vi "! SI Image TCP-IP Client 4.vi"(0 "TCP/IP Address":string="Localhost") -> ()   [LabVIEW 2015]
doc: "This is a robust TCP/IP receiver (client) vi written to work with the transmitter (server) example. This routine is designed to work in the following way:\n\n1. Runs 24/7 and waits to the server to attach to the port and starts to receive data.\n2. Senses when there is not data - but the server is running - shows that server is attached, but is waiting for data.\n3. Senses when there is no server and polls the TCP/IP port for the server to attach. Attaches to the server and begins receipt of data when server begins sending.\n3. Will not stop, quit or error unless you press the STOP button.\n\nNotes: For sub-VI use you'll need to make 2 possbile changes:\nSince this runs all the time - this will halt execution when used as a sub-VI unless \n1. Add Global Vars inside this routine and run it in a seperate loop.\n2. Simply wire the STOP button down so it only runs once.\n\n\nWritten by: Jack Hamilton\nHamilton2@aol.com\nEngineering Consulting\nLab-Useful: LabVIEW tips, Tricks and downloads\nHttp://www.lanset.com/salient1\n714-839-6375 Office (Southern California)\n\nPermission by author for free distribution"
uses:
  Client Acquisition Mode Menu.ctl
  Frame Mode 1.ctl
  CCD Format.ctl
panel:
  in  "index 3":i32=2
  in  "index 2":i32=1
  in  "index 1":i32
  in  "Set CCD Format":bool
  in  "Readout Mode":u8(ring) items=["Mode 0", "Mode 1"]
  in  "CCD Format Parameters":T1={"Serial Origin"=50, "Serial Length"=512, "Serial Binning"=1, "Parallel Origin"=0, "Parallel Length"=1024, "Parallel Binning"=1} {"Parallel Binning" min=1 max=5000 step=1; "Parallel Length" min=0 max=65535 step=1; "Parallel Origin" min=0 max=9000 step=1; "Serial Binning" min=1 max=5000 step=1; "Serial Length" min=0 max=65535 step=1; "Serial Origin" min=0 max=9000 step=1}
  in  "Save":bool
  in  "Frames":i32=1 min=1 step=1
  in  "Frame Mode":T2 items=["Single Frame Buffer", "Multiple Frame Buffer"]
  in  "Acq Mode":T3 caption="Acquisition Mode"
  in  "# to Average":u32=2 caption="of"
  out "Acquiring":u32
  in  "Save As":u16(ring) items=["U16 FITS", "I16 FITS", "I32 FITS", "SGL FITS", "U16 TIFF", "I16 TIFF", "I32 TIFF", "SGL TIFF"]
  out "P Len":i32
  out "S Len":i32
  out "Vacuum Pressure":sgl format="%.3f"
  out "Backplate Temp.":sgl format="%.1f"
  out "CCD Temp.":sgl format="%.1f"
  out "Camera Status [ ]":sgl[](array[numeric])
  out "Image Header":string
  in  "Function":T4(ring)
  in  "Perform Function":bool
  out "Function #":u16
  out "Packet\nError code":i32
  out "Image":sgl[][](graph)
  in  "RO Done":bool
  out "% Complete":u16(slide) caption="% Readout" scale=0.0..100.0
  out "% Exposure":u16(slide) scale=0.0..100.0
  in  "File Name":string
  out "TCP/IP ID":refnum<k5>
  in  "TCP/IP Mode":u16(ring)=1 items=["Retrieve Image Buffer", "Acquire and transfer to client", "Acquire and hold in Server Image Buffer", "Acquire, transfer to client and save to Server's disk", "Acquire, save to Server's disk and hold in Server Image Buffer"]
  in  "Exposure Time":dbl=0.1 min=0.0 format="%.3t"
  in  "Acq 1 Type":u16(ring) items=["Light Exposure", "Dark Exposure", "Test Image", "Triggered Acq.", "TDI Internal Paced", "TDI External Paced"]
  in  "Acquire":bool
  in  "Display Style":i32(ring)=3 items=["Normal String", "\\ Codes", "Password", "Hexdump"]
  out "Read String":string
  in  "Stop":bool
  out "Connection Status":bool
  out "Error out":errorcluster
  in  "Port":u16=2055
  # "TCP/IP Settings"
  # "Connection Status"
  # "(Use 'Localhost' for same machine)"
  # "Parallel"
  # "Serial"
  # "Origin"
  # "Length"
  # "Binning"
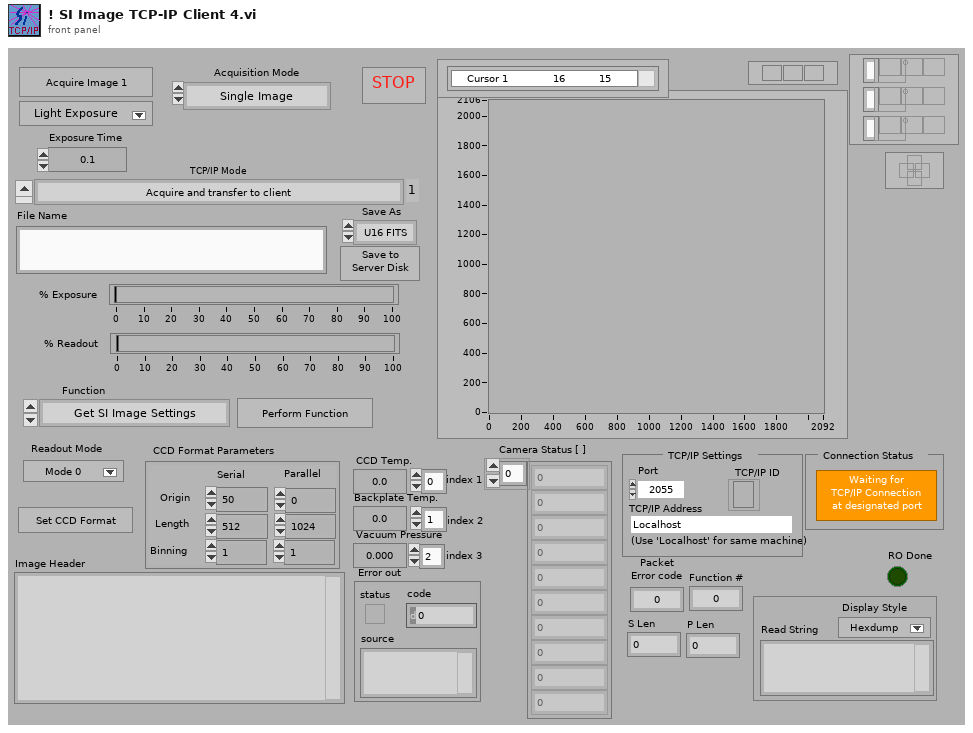
[diagram p1: front panel]
types:
  T1 = typedef "CCD Format.ctl" = cluster{"Serial Origin":i32, "Serial Length":i32, "Serial Binning":i32, "Parallel Origin":i32, "Parallel Length":i32, "Parallel Binning":i32}
  T2 = typedef "Frame Mode 1.ctl" = i32
  T3 = typedef "Client Acquisition Mode Menu.ctl" = enum16{"Single Image", "Average Images", "Multiple Frames"}
  T4 = enum16{"Get SI Image Settings", "Get Camera Status", "Get Image 1 Header", "Get Image 2 Header"}
  T5 = cluster{"% Exp.":u16, "%Readout":u16, "Relative Pos.":u32, "Acquiring":dbl}
  T6 = typedef "TCP-IP Image Packet.ctl" = cluster{"Image ID":u16, "Image Type":u16, "Serial Length":u16, "Parallel Length":u16, "# of Packets":u16, "Packet #":u16, "Offset":u32, "Image Bytes":u32, "Image Data $":string}
  T7 = typedef "SI Image Settings 1.ctl" = cluster{"Exp. Time":u32, "# of Modes":u8, "Mode #":u8, "Avg N Images":u32, "Frames":u32, "Acq. Mode":u16, "Acq. Type":u16, "Serial Origin":i32, "Serial Length":i32, "Serial Binning":i32, "Parallel Origin":i32, "Parallel Length":i32, "Parallel Binning":i32}
  T8 = cluster{"Serial Origin":i32, "Serial Length":i32, "Serial Binning":i32, "Parallel Origin":i32, "Parallel Length":i32, "Parallel Binning":i32}
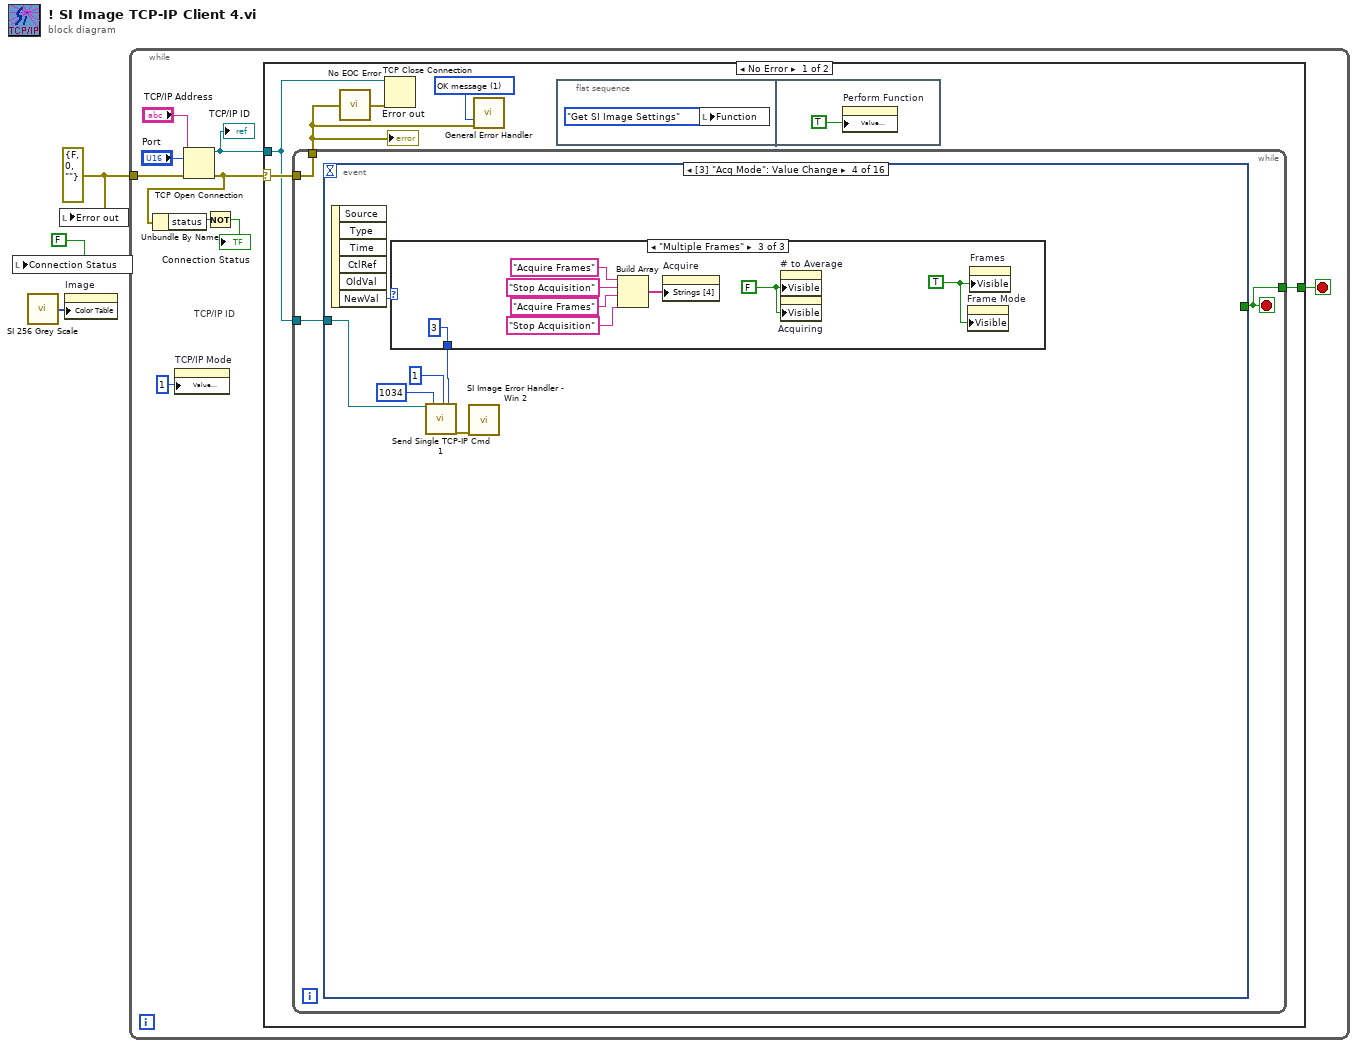
[diagram p0: block diagram]
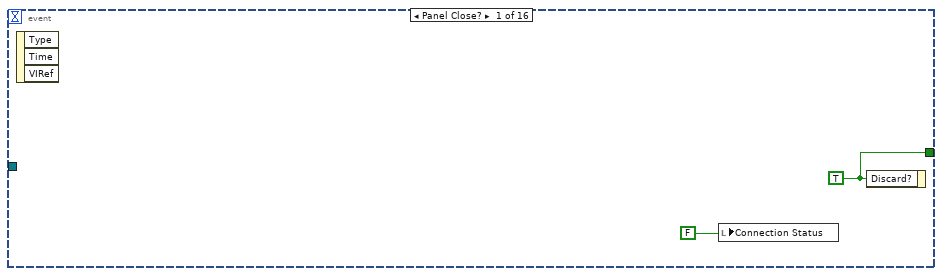
[diagram p2: hidden frame]
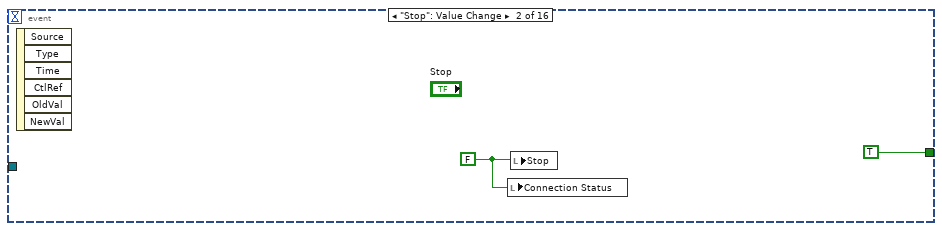
[diagram p3: hidden frame]
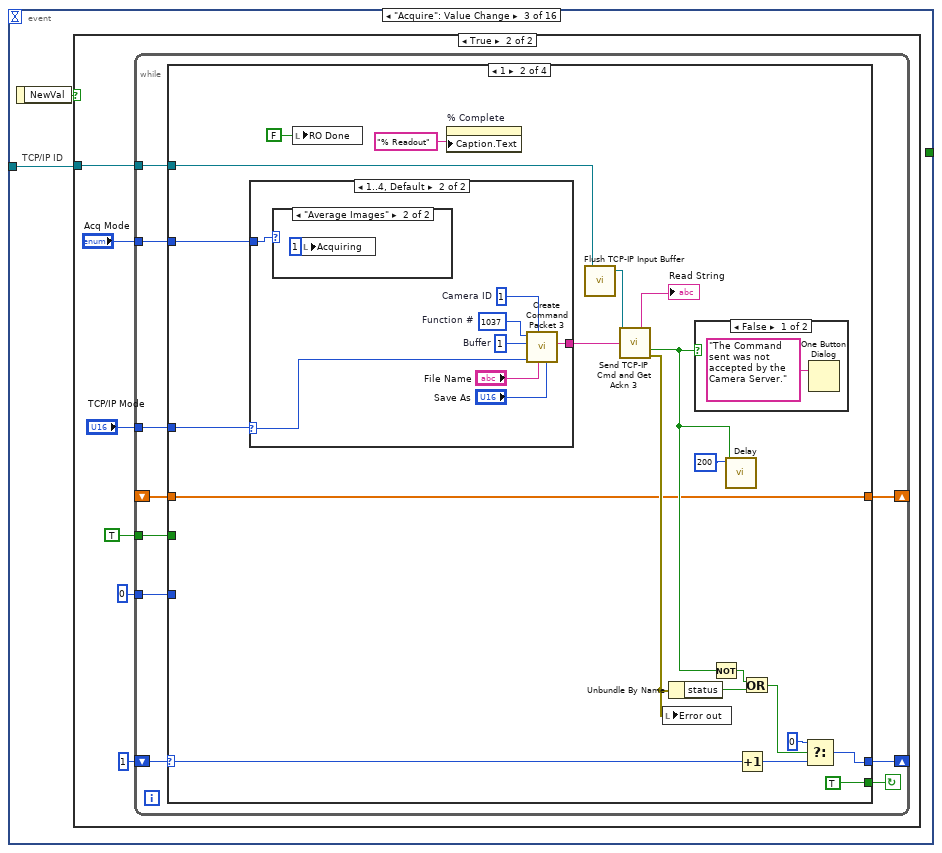
[diagram p4: hidden frame]
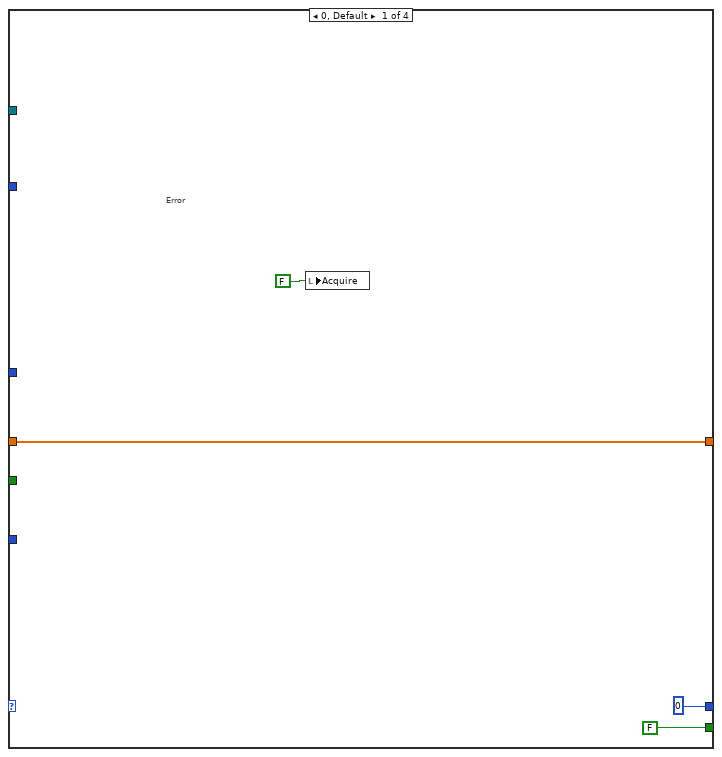
[diagram p6: hidden frame]
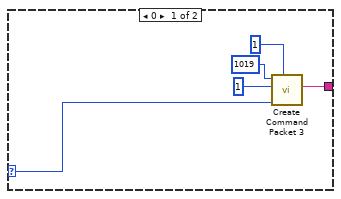
[diagram p7: hidden frame]
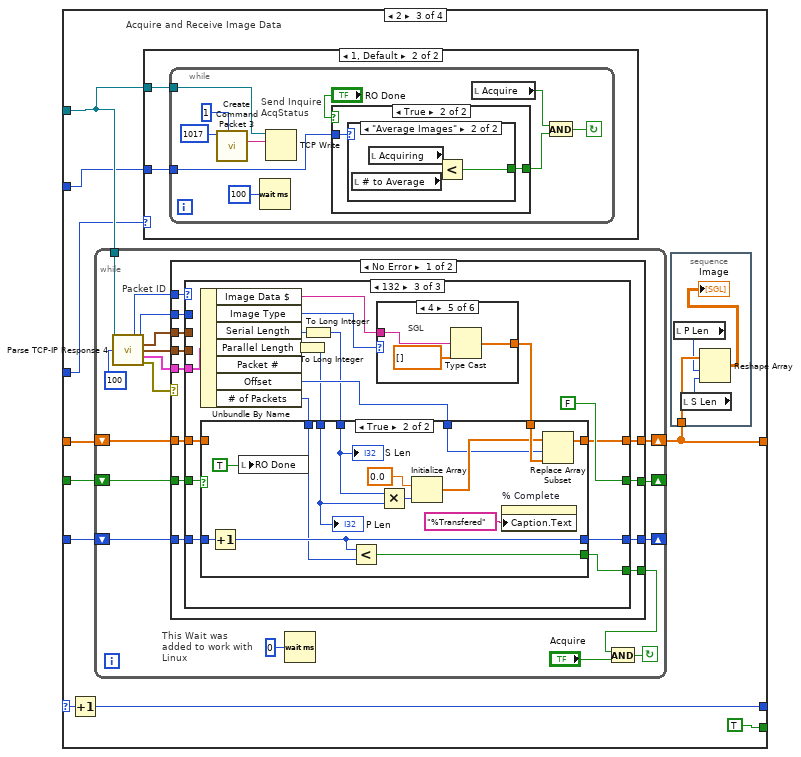
[diagram p10: hidden frame]
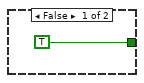
[diagram p12: hidden frame]
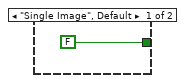
[diagram p13: hidden frame]
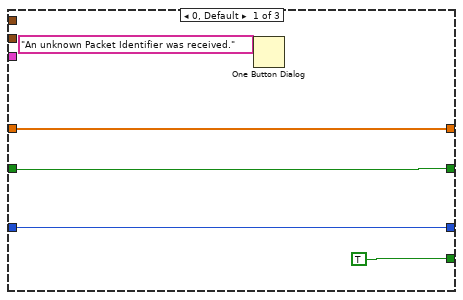
[diagram p14: hidden frame]
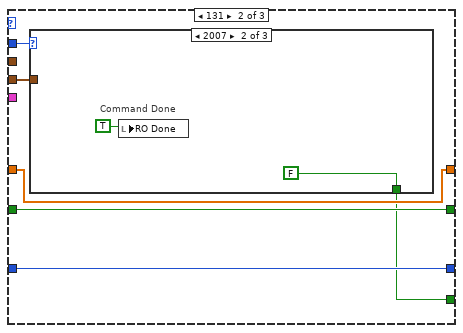
[diagram p15: hidden frame]
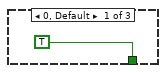
[diagram p16: hidden frame]
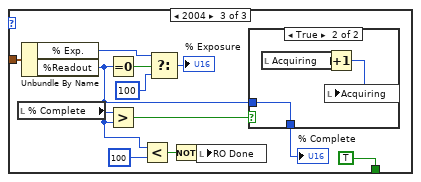
[diagram p17: hidden frame]
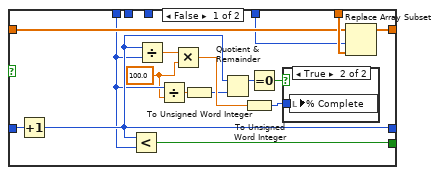
[diagram p19: hidden frame]
diagram:
  w3 = errorcluster {"status"=FALSE, "code"=0, "source"=""} ("error in (no error)")
  n1 = local write "Connection Status"(FALSE ("stop")) -> ()
  n2 = call "SI 256 Grey Scale.vi"() -> (w1:u32[])
  n3 = local write "Error out"(w3) -> ()
  n4 = property on="Image" class="IntGraph (strict)"("Color Table"=w1) -> ()  [unwired: 2 in, 2 out]
  n5 = while {
    tunnel: w3 -> [w7]
    stop <- w8 stop-if-true
    # "TCP/IP ID"
    n6 = property on="TCP/IP Mode" class="Ring (strict)"("Value (Signaling)"=u16 1) -> ()  [unwired: 2 in, 2 out]
    n7 = TCP Open Connection(address="TCP/IP Address", remote port or service name="Port", error in (no error)=w7) -> (connection ID=w12:refnum<k5>, error out=w9:errorcluster)  [unwired: 2 in]
    "TCP/IP ID" <- w12
    n8 = Unbundle By Name(w9) -> ("status"=w10:bool)
    n9 = Not(x=w10) -> (.not. x?=→"Connection Status":bool)
    n10 = case shown="No Error" w9 {
      selector: w9 -> [w17 _]
      tunnel: w12 -> [w14 _]
      tunnel: [w16 w540] -> w8
      frame No Error {
        w18 = u16 1 items=["no dialog", "OK message", "continue or stop message"] ("type of dialog (OK msg:1)")
        n11 = while {
          tunnel: [w22] -> w16
          tunnel: [w23] -> w13
          tunnel: w17 -> [w23]
          tunnel: w14 -> [w21]
          stop <- w22 stop-if-true
          n12 = event shown="[3] \"Acq Mode\": Value Change" {
            selector: _ -> [_ _ _ _ _ _ _ _ _ _ _ _ _ _ _ _]
            dyn-events: _ -> [_ _ _ _ _ _ _ _ _ _ _ _ _ _ _ _]
            timeout: _ -> [_ _ _ _ _ _ _ _ _ _ _ _ _ _ _ _]
            tunnel: [w25 TRUE _ _ _ _ _ _ _ _ _ _ _ _ _ _] -> w22
            tunnel: w21 -> [_ _ w28 w295 w330 w336 w344 w349 w354 w360 w366 w372 _ w415 _ _]
            event Panel Close? {
              w25 = TRUE ("Discard?")
              n13 = event-data() -> ()  [unwired: 1 in, 3 out]
              n14 = local write "Connection Status"(FALSE ("stop")) -> ()
              n15 = event-data("Discard?"=w25) -> ()  [unwired: 1 in, 1 out]
            }
            event "Stop": Value Change {
              w26 = FALSE ("Stop")
              n16 = event-data() -> ()  [unwired: 1 in, 6 out]
              n17 = local write "Connection Status"(w26) -> ()
              n18 = local write "Stop"(w26) -> ()
            }
            event "Acquire": Value Change {
              # "TCP/IP ID"
              n19 = event-data() -> ("NewVal"=w29:bool)  [unwired: 1 in]
              n20 = case shown="True" w29 {
                tunnel: w28 -> [_ w34]
                frame False {
                }
                frame True {
                  n21 = while {
                    tunnel: u16 0 -> [w37]
                    tunnel: TRUE -> [w38]
                    shift-left: _ -> [w40]
                    shift-right: [w39] -> _
                    tunnel: w34 -> [w41]
                    tunnel: "TCP/IP Mode" -> [w42]
                    shift-left: 1 -> [w45]
                    shift-right: [w44] -> _
                    tunnel: "Acq Mode" -> [w36]
                    stop <- w43 continue-if-true
                    n22 = case shown="1" w45 {
                      selector: w45 -> [_ w69 w93 w268]
                      tunnel: [0 w61 w94 w268] -> w44
                      tunnel: [FALSE TRUE TRUE w263] -> w43
                      tunnel: w42 -> [_ w55 w85 w266]
                      tunnel: w41 -> [_ w67 w91 w267]
                      tunnel: w40 -> [w46 w51 w90 w262]
                      tunnel: [w46 w51 w87 w262] -> w39
                      tunnel: w38 -> [_ _ w89 _]
                      tunnel: w37 -> [_ _ w88 _]
                      tunnel: w36 -> [_ w50 w86 w261]
                      frame 0, Default {
                        # "Error"
                        n23 = local write "Acquire"(FALSE) -> ()
                      }
                      frame 1 {
                        n24 = case shown="1..4, Default" w55 {
                          selector: w55 -> [w71 w78]
                          tunnel: [w72 w80] -> w65
                          tunnel: w50 -> [_ w75]
                          frame 0 {
                            n25 = call "Create Command Packet 3.vi"("Camera ID (1)"=u8 1 ("Camera ID"), "Mode"=w71, "Buffer/Avg #/Frames"=u16 1 ("Buffer #"), "Function #"=u16 1019) -> ("Cmd Packet"=w72:string)  [unwired: 7 in]
                          }
                          frame 1..4, Default {
                            w82 = u16 1037  # Function #
                            w79 = u32 1  # Buffer
                            w81 = u8 1  # Camera ID
                            n26 = case shown="\"Average Images\"" w75 {
                              frame "Single Image", Default {
                              }
                              frame "Average Images" {
                                n27 = local write "Acquiring"(u32 1 ("Acquiring")) -> ()
                              }
                            }
                            n28 = call "Create Command Packet 3.vi"("Save As"="Save As", "File Name"="File Name", "Camera ID (1)"=w81, "Mode"=w78, "Buffer/Avg #/Frames"=w79, "Function #"=w82) -> ("Cmd Packet"=w80:string)  [unwired: 5 in]
                          }
                        }
                        n29 = local write "RO Done"(FALSE ("RO Done")) -> ()
                        n30 = property on="% Complete" class="Slide (strict)"("Caption.Text"="% Readout") -> ()  [unwired: 2 in, 2 out]
                        n31 = call "Flush TCP-IP Input Buffer.vi"("TCP/IP ID"=w67) -> ("TCP/IP ID Out"=w66:refnum<k5>)  [unwired: 4 in]
                        n32 = call "Send TCP-IP Cmd and Get Ackn 3.vi"("TCP/IP ID In"=w66, "Cmd Packet"=w65) -> ("Read String"=→"Read String":string, "Accepted Flag"=w57:bool, "error out"=w52:errorcluster)  [unwired: 7 in, 4 out]
                        n33 = local write "Error out"(w52) -> ()
                        n34 = Unbundle By Name(w52) -> ("status"=w64:bool)
                        n35 = case shown="False" w57 {
                          frame False {
                            n36 = One Button Dialog(message="The Command sent was not accepted by the Camera Server.") -> ()  [unwired: 1 in, 1 out]
                          }
                          frame True {
                          }
                        }
                        n37 = Not(x=w57) -> (.not. x?=w59:bool)
                        n38 = call "Delay.vi"("Boolean In"=w57, "milliseconds to wait (10)"=u32 200) -> ()  [unwired: 8 in, 2 out]
                        n39 = Increment(x=w69) -> (x+1=w63:i32)
                        n40 = Or(x=w59, y=w64) -> (x .or. y?=w60:bool)
                        n41 = Select(t=0, s=w60, f=w63) -> (s? t:f=w61:i32)
                      }
                      frame 2 {
                        # "Acquire and Receive Image Data"
                        n42 = Increment(x=w93) -> (x+1=w94:i32)
                        n43 = while {
                          shift-left: w88 -> [w119]
                          shift-right: [w118] -> _
                          shift-left: w89 -> [w121]
                          shift-right: [w120] -> _
                          shift-left: w90 -> [w122]
                          shift-right: [w116] -> w87
                          tunnel: w91 -> [w131]
                          stop <- w127 continue-if-true
                          # "This Wait was added to work with Linux"
                          # "Packet ID"
                          n44 = call "Parse TCP-IP Response 4.vi"("TCP/IP ID"=w131, "timeout ms (5000)"=100) -> ("Packet ID"=w130:u8, "Data Type"=w124:u16, "Command Done"=w129:cluster{"Function #":u16}, "Acq. Status"=w128:T5, "Image Packet"=w123:T6, "error out"=w125:errorcluster)  [unwired: 3 in, 5 out]
                          n45 = case shown="No Error" w125 {
                            selector: w125 -> [_ w246]
                            tunnel: w130 -> [w143 _]
                            tunnel: w129 -> [w142 _]
                            tunnel: w128 -> [w141 _]
                            tunnel: [w140 w247] -> w126
                            tunnel: w124 -> [w139 _]
                            tunnel: w123 -> [w138 _]
                            tunnel: w122 -> [w137 w250]
                            tunnel: [w136 w250] -> w116
                            tunnel: w121 -> [w135 w251]
                            tunnel: [w134 w251] -> w120
                            tunnel: w119 -> [w133 w249]
                            tunnel: [w132 w249] -> w118
                            frame No Error {
                              n46 = case shown="132" w143 {
                                tunnel: w142 -> [_ _ _]
                                tunnel: w141 -> [_ w154 _]
                                tunnel: [TRUE w149 w179] -> w140
                                tunnel: w139 -> [_ w151 _]
                                tunnel: w138 -> [_ _ w187]
                                tunnel: w137 -> [w144 w150 w178]
                                tunnel: [w144 w150 w182] -> w136
                                tunnel: w135 -> [w147 w153 w177]
                                tunnel: [w147 w153 FALSE] -> w134
                                tunnel: w133 -> [w146 w152 w181]
                                tunnel: [w146 w152 w180] -> w132
                                frame 0, Default {
                                n47 = One Button Dialog(message="An unknown Packet Identifier was received.") -> ()  [unwired: 1 in, 1 out]
                                }
                                frame 131 {
                                n48 = case shown="2007" w151 {
                                tunnel: w154 -> [_ _ w170]
                                tunnel: [TRUE FALSE TRUE] -> w149
                                frame 0, Default {
                                }
                                frame 2007 {
                                # "Command Done"
                                n49 = local write "RO Done"(TRUE) -> ()
                                }
                                frame 2004 {
                                n50 = local read "% Complete"() -> (w164:u16)
                                n51 = Unbundle By Name(w170) -> ("% Exp."=w159:u16, "%Readout"=w162:u16)
                                n52 = Equal To 0?(x=w162) -> (x = 0?=w161:bool)
                                n53 = Greater?(x=w164, y=w162) -> (0:w163:bool)
                                n54 = Less?(x=w162, y=u16 100) -> (x < y?=w168:bool)
                                n55 = Select(t=w159, s=w161, f=u16 100) -> (s? t:f=→"% Exposure":u16)
                                n56 = Not(x=w168) -> (.not. x?=w167:bool)
                                n57 = local write "RO Done"(w167) -> ()
                                n58 = case shown="True" w163 {
                                tunnel: [w171 w172] -> w165
                                tunnel: w162 -> [w171 w172]
                                frame False {
                                }
                                frame True {
                                n59 = local read "Acquiring"() -> (w173:u32)
                                n60 = Increment(x=w173) -> (x+1=w174:u32)
                                n61 = local write "Acquiring"(w174) -> ()
                                }
                                }
                                "% Complete" <- w165
                                }
                                }
                                }
                                frame 132 {
                                n62 = Unbundle By Name(w187) -> ("Image Data $"=w190:string, "Image Type"=w189:u16, "Serial Length"=w186:u16, "Parallel Length"=w185:u16, "Offset"=w184:u32, "# of Packets"=w188:u16)  [unwired: 1 out]
                                n63 = To Long Integer(number=w185) -> (32bit integer=w175:i32)
                                n64 = To Long Integer(number=w186) -> (32bit integer=w176:i32)
                                n65 = case shown="4" w189 {
                                tunnel: [w225 w228 w233 w236 w240 w243] -> w183
                                tunnel: w190 -> [w223 w227 w231 w235 w239 w242]
                                frame 0, Default {
                                # "U16"
                                n66 = Type Cast(type=u16[] [] ("Array Constant"), x=w223) -> (*(type *) &x=w226:u16[])
                                n67 = To Single Precision Float(number=w226) -> (single precision float=w225:sgl[])
                                }
                                frame 1 {
                                # "I16"
                                n68 = Type Cast(type=i16[] [] ("Array Constant"), x=w227) -> (*(type *) &x=w230:i16[])
                                n69 = To Single Precision Float(number=w230) -> (single precision float=w228:sgl[])
                                }
                                frame 2 {
                                # "U32"
                                n70 = Type Cast(type=u32[] [] ("Array Constant"), x=w231) -> (*(type *) &x=w234:u32[])
                                n71 = To Single Precision Float(number=w234) -> (single precision float=w233:sgl[])
                                }
                                frame 3 {
                                # "I32"
                                n72 = Type Cast(type=i32[] [] ("Array Constant"), x=w235) -> (*(type *) &x=w238:i32[])
                                n73 = To Single Precision Float(number=w238) -> (single precision float=w236:sgl[])
                                }
                                frame 4 {
                                # "SGL"
                                n74 = Type Cast(type=sgl[] [] ("Array Constant"), x=w239) -> (*(type *) &x=w240:sgl[])
                                }
                                frame 5 {
                                # "DBL"
                                n75 = Type Cast(type=dbl[] [] ("Array Constant"), x=w242) -> (*(type *) &x=w245:dbl[])
                                n76 = To Single Precision Float(number=w245) -> (single precision float=w243:sgl[])
                                }
                                }
                                n77 = case shown="True" w177 {
                                tunnel: w178 -> [w198 _]
                                tunnel: w176 -> [_ w210]
                                tunnel: w175 -> [_ w209]
                                tunnel: [w199 w221] -> w182
                                tunnel: w183 -> [w207 w220]
                                tunnel: w181 -> [w206 w218]
                                tunnel: [w196 w217] -> w180
                                tunnel: [w205 w216] -> w179
                                tunnel: w184 -> [w197 w213]
                                tunnel: w188 -> [w194 w212]
                                frame False {
                                w193 = 100.0 ("y")
                                n78 = Increment(x=w206) -> (x+1=w196:u16)
                                n79 = Less?(x=w196, y=w194) -> (x < y?=w205:bool)
                                n80 = Divide(x=w196, y=w194) -> (x/y=w201:dbl)
                                n81 = Divide(x=w194, y=w193) -> (x/y=w195:dbl)
                                n82 = Multiply(x=w201, y=w193) -> (x*y=w200:dbl)
                                n83 = To Unsigned Word Integer(number=w195) -> (unsigned 16bit integer=w192:u16)
                                n84 = Quotient & Remainder(x=w196, y=w192) -> (x-y*floor(x/y)=w204:u16)  [unwired: 1 out]
                                n85 = To Unsigned Word Integer(number=w200) -> (unsigned 16bit integer=w202:u16)
                                n86 = Equal To 0?(x=w204) -> (x = 0?=w203:bool)
                                n87 = case shown="True" w203 {
                                tunnel: w202 -> [_ w208]
                                frame False {
                                }
                                frame True {
                                n88 = local write "% Complete"(w208) -> ()
                                }
                                }
                                n89 = Replace Array Subset(array=w198, new element=w207, index=w197) -> (w199:sgl[])
                                }
                                frame True {
                                n90 = Increment(x=w218) -> (x+1=w217:u16)
                                n91 = local write "RO Done"(TRUE) -> ()
                                n92 = Less?(x=w217, y=w212) -> (x < y?=w216:bool)
                                n93 = Multiply(x=w210, y=w209) -> (x*y=w214:i32)
                                n94 = Initialize Array(sgl 0.0 ("Element Data"), w214) -> (w219:sgl[])
                                n95 = property on="% Complete" class="Slide (strict)"("Caption.Text"="%Transfered") -> ()  [unwired: 2 in, 2 out]
                                n96 = Replace Array Subset(array=w219, new element=w220, index=w213) -> (w221:sgl[])
                                "S Len" <- w210
                                "P Len" <- w209
                                }
                                }
                                }
                              }
                            }
                            frame Error {
                              n97 = Unbundle By Name(w246) -> ("code"=w248:i32)
                              n98 = case shown="0, Default" w248 {
                                tunnel: w246 -> [w255 _]
                                tunnel: [w253 TRUE] -> w247
                                frame 0, Default {
                                w253 = FALSE
                                n99 = call <vilib>:"Simple Error Handler.vi"("error source (\" \")"="There was an error in a TCP/IP read during an Image Acquisition.", "error in (no error)"=w255) -> ("error out"=w252:errorcluster)  [unwired: 3 in, 4 out]
                                n100 = local write "Error out"(w252) -> ()
                                n101 = local write "Acquire"(w253) -> ()
                                }
                                frame 56 {
                                # "Timeout -  Keep going"
                                }
                              }
                            }
                          }
                          n102 = Wait (ms)(milliseconds to wait=u32 0) -> ()  [unwired: 1 out]
                          n103 = And(x=w126, y="Acquire") -> (x .and. y?=w127:bool)
                        }
                        n104 = case shown="1, Default" w85 {
                          tunnel: w91 -> [_ w96]
                          tunnel: w86 -> [_ w95]
                          frame 0 {
                          }
                          frame 1, Default {
                            n105 = while {
                              tunnel: w96 -> [w103]
                              tunnel: w95 -> [w97]
                              stop <- w101 continue-if-true
                              # "Send Inquire\nAcqStatus"
                              n106 = call "Create Command Packet 3.vi"("Camera ID (1)"=u8 1 ("Camera ID"), "Function #"=u16 1017) -> ("Cmd Packet"=w104:string)  [unwired: 9 in]
                              n107 = Wait (ms)(milliseconds to wait=u32 100) -> ()  [unwired: 1 out]
                              n108 = TCP Write(connection ID=w103, data in=w104) -> ()  [unwired: 2 in, 3 out]
                              n109 = case shown="True" "RO Done" {
                                tunnel: [TRUE w109] -> w100
                                tunnel: w97 -> [_ w108]
                                frame False {
                                }
                                frame True {
                                n110 = case shown="\"Average Images\"" w108 {
                                tunnel: [FALSE w111] -> w109
                                frame "Single Image", Default {
                                }
                                frame "Average Images" {
                                n111 = local read "# to Average"() -> (w112:u32)
                                n112 = local read "Acquiring"() -> (w113:u32)
                                n113 = Less?(x=w113, y=w112) -> (x < y?=w111:bool)
                                }
                                }
                                }
                              }
                              n114 = local read "Acquire"() -> (w98:bool)
                              n115 = And(x=w98, y=w100) -> (x .and. y?=w101:bool)
                            }
                          }
                        }
                        n116 = stacked-sequence {
                          tunnel: w87 -> [w260]
                          frame #0 {
                            n117 = local read "P Len"() -> (w259:i32)
                            n118 = local read "S Len"() -> (w258:i32)
                            n119 = Reshape Array(w260, w259, w258) -> (→"Image":sgl[][])
                          }
                        }
                      }
                      frame 3 {
                        w263 = FALSE
                        n120 = case shown="1, Default" w266 {
                          selector: w266 -> [w270 w279 w293]
                          tunnel: w267 -> [_ w280 _]
                          tunnel: [w270 w279 w293] -> w264
                          tunnel: w261 -> [_ w273 _]
                          frame 0 {
                          }
                          frame 1, Default {
                            # "If Exposure was not 100%, acquisition was terminated so send TerminateAcquisition command."
                            n121 = Equal?(x=w273, y=Client_Acquisition_Mode_Menu."Average Images") -> (x = y?=w271:bool)
                            n122 = local read "# to Average"() -> (w277:u32)
                            n123 = local read "% Exposure"() -> (w282:u16)
                            n124 = local read "Acquiring"() -> (w278:u32)
                            n125 = Less?(x=w278, y=w277) -> (x < y?=w276:bool)
                            n126 = Less?(x=w282, y=u16 100) -> (x < y?=w275:bool)
                            n127 = Select(t=w276, s=w271, f=w275) -> (s? t:f=w274:bool)
                            n128 = case shown="True" w274 {
                              tunnel: w280 -> [_ w291]
                              frame False {
                              }
                              frame True {
                                n129 = call "Create Command Packet 3.vi"("Camera ID (1)"=u8 1 ("Camera ID"), "Function #"=u16 1018) -> ("Cmd Packet"=w289:string)  [unwired: 9 in]
                                n130 = call "Flush TCP-IP Input Buffer.vi"("TCP/IP ID"=w291) -> ("TCP/IP ID Out"=w285:refnum<k5>)  [unwired: 4 in]
                                n131 = TCP Write(connection ID=w285, data in=w289) -> (error out=w288:errorcluster)  [unwired: 2 in, 2 out]
                                n132 = call "Parse TCP-IP Response 4.vi"("TCP/IP ID"=w285, "error in (no error)"=w288) -> ("Packet Error Code"=→"Packet\nError code":i32, "Command Done"=w287:cluster{"Function #":u16}, "error out"=w283:errorcluster)  [unwired: 3 in, 8 out]
                                n133 = Unbundle By Name(w287) -> ("Function #"=→"Function #":u16)
                                n134 = local write "Error out"(w283) -> ()
                              }
                            }
                          }
                          frame 5 {
                          }
                        }
                        n135 = stacked-sequence {
                          tunnel: w264 -> [_]
                          frame #0 {
                            w269 = u16 0 ("% Exposure")
                            n136 = local write "% Exposure"(w269) -> ()
                            n137 = local write "% Complete"(w269) -> ()
                            "Acquiring" <- w269
                          }
                        }
                        n138 = property on="% Complete" class="Slide (strict)"("Caption.Text"="% Readout") -> ()  [unwired: 2 in, 2 out]
                        n139 = local write "Acquire"(w263) -> ()
                      }
                    }
                  }
                }
              }
            }
            event Value Change {
              n140 = event-data() -> ("NewVal"=w299:T3)  [unwired: 1 in, 5 out]
              n141 = case shown="\"Multiple Frames\"" w299 {
                selector: w299 -> [w301 w310 _]
                tunnel: [w300 w309 u8 3 ("Acq. Mode/Type/Buffer")] -> w294
                frame "Single Image", Default {
                  w302 = FALSE ("Visible")
                  w303 = FALSE ("Visible")
                  n142 = To Unsigned Byte Integer(number=w301) -> (unsigned 8bit integer=w300:u8)
                  n143 = Build Array("Acquire Image 1", "Stop Acquisition", "Acquire Image 1", "Stop Acquisition") -> (w304:string[])
                  n144 = property on="Acquire" class="Bool (strict)"("Strings [4]"=w304) -> ()  [unwired: 2 in, 2 out]
                  n145 = property on="# to Average" class="DigNum (strict)"("Visible"=w302) -> ()  [unwired: 2 in, 2 out]
                  n146 = property on="Acquiring" class="DigNum (strict)"("Visible"=w302) -> ()  [unwired: 2 in, 2 out]
                  n147 = property on="Frames" class="DigNum (strict)"("Visible"=w303) -> ()  [unwired: 2 in, 2 out]
                  n148 = property on="Frame Mode" class="Ring (strict)"("Visible"=w303) -> ()  [unwired: 2 in, 2 out]
                }
                frame "Average Images" {
                  w311 = TRUE ("Visible")
                  w312 = FALSE ("Visible")
                  n149 = To Unsigned Byte Integer(number=w310) -> (unsigned 8bit integer=w309:u8)
                  n150 = Build Array("Acquire Average", "Stop Acquisition", "Acquire Average", "Stop Acquisition") -> (w313:string[])
                  n151 = property on="Acquire" class="Bool (strict)"("Strings [4]"=w313) -> ()  [unwired: 2 in, 2 out]
                  n152 = property on="# to Average" class="DigNum (strict)"("Visible"=w311) -> ()  [unwired: 2 in, 2 out]
                  n153 = property on="Acquiring" class="DigNum (strict)"("Visible"=w311) -> ()  [unwired: 2 in, 2 out]
                  n154 = property on="Frame Mode" class="Ring (strict)"("Visible"=w312) -> ()  [unwired: 2 in, 2 out]
                  n155 = property on="Frames" class="DigNum (strict)"("Visible"=w312) -> ()  [unwired: 2 in, 2 out]
                }
                frame "Multiple Frames" {
                  w319 = FALSE ("Visible")
                  w320 = TRUE ("Visible")
                  n156 = Build Array("Acquire Frames", "Stop Acquisition", "Acquire Frames", "Stop Acquisition") -> (w321:string[])
                  n157 = property on="Acquire" class="Bool (strict)"("Strings [4]"=w321) -> ()  [unwired: 2 in, 2 out]
                  n158 = property on="# to Average" class="DigNum (strict)"("Visible"=w319) -> ()  [unwired: 2 in, 2 out]
                  n159 = property on="Acquiring" class="DigNum (strict)"("Visible"=w319) -> ()  [unwired: 2 in, 2 out]
                  n160 = property on="Frame Mode" class="Ring (strict)"("Visible"=w320) -> ()  [unwired: 2 in, 2 out]
                  n161 = property on="Frames" class="DigNum (strict)"("Visible"=w320) -> ()  [unwired: 2 in, 2 out]
                }
              }
              n162 = call "Send Single TCP-IP Cmd 1.vi"("TCP/IP ID"=w295, "Function #"=u16 1034, "Camera ID"=u8 1, "Acq. Mode/Type/Frame Mode/RO Mode #"=w294) -> ("Error Out"=w296:errorcluster)  [unwired: 12 in, 3 out]
              n163 = call "SI Image Error Handler - Win 2.vi"("error in (no error)"=w296) -> ()  [unwired: 4 in, 1 out]
            }
            event "Exposure Time": Value Change {
              # "ET in ms"
              n164 = event-data() -> ("NewVal"=w327:dbl)  [unwired: 1 in, 5 out]
              n165 = Multiply(x=w327, y=1000.0) -> (x*y=w328:dbl)
              n166 = To Unsigned Long Integer(number=w328) -> (unsigned 32bit integer=w326:u32)
              n167 = call "Send Single TCP-IP Cmd 1.vi"("TCP/IP ID"=w330, "Exposure Time (ms)"=w326, "Function #"=u16 1035, "Camera ID"=u8 1) -> ("Error Out"=w331:errorcluster)  [unwired: 12 in, 3 out]
              n168 = call "SI Image Error Handler - Win 2.vi"("error in (no error)"=w331) -> ()  [unwired: 4 in, 1 out]
            }
            event "Readout Mode": Value Change {
              n169 = event-data() -> ("NewVal"=w335:u8)  [unwired: 1 in, 3 out]
              n170 = call "Send Single TCP-IP Cmd 1.vi"("TCP/IP ID"=w336, "Function #"=u16 1042, "Camera ID"=u8 1, "Acq. Mode/Type/Frame Mode/RO Mode #"=w335) -> ("Error Out"=w337:errorcluster)  [unwired: 12 in, 3 out]
              n171 = call "SI Image Error Handler - Win 2.vi"("error in (no error)"=w337) -> ("error out"=w334:errorcluster)  [unwired: 4 in]
              n172 = flat-sequence {
                tunnel: w334 -> [_]
                frame #0 {
                  n173 = local write "Function"(T4."Get SI Image Settings" ("Function")) -> ()
                }
                frame #1 {
                  n174 = property on="Perform Function" class="Bool (strict)"("Value (Signaling)"=TRUE) -> ()  [unwired: 2 in, 2 out]
                }
              }
            }
            event "Acq 1 Type": Value Change {
              n175 = event-data() -> ("NewVal"=w343:u16)  [unwired: 1 in, 5 out]
              n176 = call "Send Single TCP-IP Cmd 1.vi"("TCP/IP ID"=w344, "Buffer/Avg #/Frames"=u16 1, "Function #"=u16 1036, "Camera ID"=u8 1, "Acq. Mode/Type/Frame Mode/RO Mode #"=w343) -> ("Error Out"=w345:errorcluster)  [unwired: 11 in, 3 out]
              n177 = call "SI Image Error Handler - Win 2.vi"("error in (no error)"=w345) -> ()  [unwired: 4 in, 1 out]
            }
            event Value Change {
              n178 = event-data() -> ("NewVal"=w348:T2)  [unwired: 1 in, 5 out]
              n179 = call "Send Single TCP-IP Cmd 1.vi"("TCP/IP ID"=w349, "Function #"=u16 1040, "Camera ID"=u8 1, "Acq. Mode/Type/Frame Mode/RO Mode #"=w348) -> ("Error Out"=w350:errorcluster)  [unwired: 12 in, 3 out]
              n180 = call "SI Image Error Handler - Win 2.vi"("error in (no error)"=w350) -> ()  [unwired: 4 in, 1 out]
            }
            event "Frames": Value Change {
              n181 = event-data() -> ("NewVal"=w353:i32)  [unwired: 1 in, 5 out]
              n182 = call "Send Single TCP-IP Cmd 1.vi"("TCP/IP ID"=w354, "Buffer/Avg #/Frames"=w353, "Function #"=u16 1039, "Camera ID"=u8 1) -> ("Error Out"=w355:errorcluster)  [unwired: 12 in, 3 out]
              n183 = call "SI Image Error Handler - Win 2.vi"("error in (no error)"=w355) -> ()  [unwired: 4 in, 1 out]
            }
            event "Set CCD Format": Value Change {
              n184 = event-data() -> ()  [unwired: 1 in, 6 out]
              n185 = call "Send Single TCP-IP Cmd 1.vi"("TCP/IP ID"=w360, "Function #"=u16 1043, "Camera ID"=u8 1, "CCD Format Parameters"="CCD Format Parameters") -> ("Error Out"=w361:errorcluster)  [unwired: 12 in, 3 out]
              n186 = call "SI Image Error Handler - Win 2.vi"("error in (no error)"=w361) -> ("error out"=w358:errorcluster)  [unwired: 4 in]
              n187 = stacked-sequence {
                tunnel: w358 -> [_]
                frame #0 {
                  n188 = local write "Set CCD Format"(FALSE ("Set CCD Format")) -> ()
                }
              }
            }
            event "# to Average": Value Change {
              n189 = event-data() -> ("NewVal"=w365:u32)  [unwired: 1 in, 5 out]
              n190 = call "Send Single TCP-IP Cmd 1.vi"("TCP/IP ID"=w366, "Buffer/Avg #/Frames"=w365, "Function #"=u16 1038, "Camera ID"=u8 1) -> ("Error Out"=w367:errorcluster)  [unwired: 12 in, 3 out]
              n191 = call "SI Image Error Handler - Win 2.vi"("error in (no error)"=w367) -> ()  [unwired: 4 in, 1 out]
            }
            event "Save": Value Change {
              n192 = event-data() -> ("NewVal"=w371:bool)  [unwired: 1 in, 5 out]
              n193 = case shown="True" w371 {
                tunnel: w372 -> [_ w378]
                tunnel: [_ w374] -> w370
                frame False {
                }
                frame True {
                  n194 = local read "File Name"() -> (w376:string)
                  n195 = local read "Save As"() -> (w375:u16)
                  n196 = call "Send Single TCP-IP Cmd 1.vi"("TCP/IP ID"=w378, "Buffer/Avg #/Frames"=u16 1, "Function #"=u16 1031, "File Name"=w376, "Camera ID"=u8 1, "Save As"=w375) -> ("Error Out"=w379:errorcluster)  [unwired: 10 in, 3 out]
                  n197 = call "SI Image Error Handler - Win 2.vi"("error in (no error)"=w379) -> ("error out"=w374:errorcluster)  [unwired: 4 in]
                }
              }
              n198 = stacked-sequence {
                tunnel: w370 -> [_]
                frame #0 {
                  n199 = local write "Save"(FALSE ("Save")) -> ()
                }
              }
            }
            event "TCP/IP Mode": Value Change {
              n200 = event-data() -> ("NewVal"=w382:u16)  [unwired: 1 in, 5 out]
              n201 = case shown="1, Default" w382 {
                frame 0 {
                  w383 = FALSE ("Visible")
                  w384 = FALSE ("Visible")
                  w385 = FALSE ("Visible")
                  n202 = Build Array("Retrieve Image", "Retrieving", "Acquire Frames", "Retrieving") -> (w386:string[])
                  n203 = property on="Acquire" class="Bool (strict)"("Strings [4]"=w386) -> ()  [unwired: 2 in, 2 out]
                  n204 = property on="Acq Mode" class="Enum (strict)"("Visible"=w383) -> ()  [unwired: 2 in, 2 out]
                  n205 = property on="Acq 1 Type" class="Ring (strict)"("Visible"=w383) -> ()  [unwired: 2 in, 2 out]
                  n206 = property on="# to Average" class="DigNum (strict)"("Visible"=w384) -> ()  [unwired: 2 in, 2 out]
                  n207 = property on="Acquiring" class="DigNum (strict)"("Visible"=w384) -> ()  [unwired: 2 in, 2 out]
                  n208 = property on="Frames" class="DigNum (strict)"("Visible"=w385) -> ()  [unwired: 2 in, 2 out]
                  n209 = property on="Frame Mode" class="Ring (strict)"("Visible"=w385) -> ()  [unwired: 2 in, 2 out]
                }
                frame 1, Default {
                  w391 = TRUE ("Visible")
                  n210 = local read "Acq Mode"() -> (w392:T3)
                  n211 = case shown="\"Single Image\", Default" w392 {
                    frame "Single Image", Default {
                      w393 = FALSE ("Visible")
                      w394 = FALSE ("Visible")
                      n212 = Build Array("Acquire Image 1", "Stop Acquisition", "Acquire Image 1", "Stop Acquisition") -> (w395:string[])
                      n213 = property on="Acquire" class="Bool (strict)"("Strings [4]"=w395) -> ()  [unwired: 2 in, 2 out]
                      n214 = property on="# to Average" class="DigNum (strict)"("Visible"=w393) -> ()  [unwired: 2 in, 2 out]
                      n215 = property on="Acquiring" class="DigNum (strict)"("Visible"=w393) -> ()  [unwired: 2 in, 2 out]
                      n216 = property on="Frame Mode" class="Ring (strict)"("Visible"=w394) -> ()  [unwired: 2 in, 2 out]
                      n217 = property on="Frames" class="DigNum (strict)"("Visible"=w394) -> ()  [unwired: 2 in, 2 out]
                    }
                    frame "Average Images" {
                      w400 = TRUE ("Visible")
                      w401 = FALSE ("Visible")
                      n218 = Build Array("Acquire Average", "Stop Acquisition", "Acquire Average", "Stop Acquisition") -> (w402:string[])
                      n219 = property on="Acquire" class="Bool (strict)"("Strings [4]"=w402) -> ()  [unwired: 2 in, 2 out]
                      n220 = property on="# to Average" class="DigNum (strict)"("Visible"=w400) -> ()  [unwired: 2 in, 2 out]
                      n221 = property on="Acquiring" class="DigNum (strict)"("Visible"=w400) -> ()  [unwired: 2 in, 2 out]
                      n222 = property on="Frame Mode" class="Ring (strict)"("Visible"=w401) -> ()  [unwired: 2 in, 2 out]
                      n223 = property on="Frames" class="DigNum (strict)"("Visible"=w401) -> ()  [unwired: 2 in, 2 out]
                    }
                    frame "Multiple Frames" {
                      w407 = FALSE ("Visible")
                      w408 = TRUE ("Visible")
                      n224 = Build Array("Acquire Frames", "Stop Acquisition", "Acquire Frames", "Stop Acquisition") -> (w409:string[])
                      n225 = property on="Acquire" class="Bool (strict)"("Strings [4]"=w409) -> ()  [unwired: 2 in, 2 out]
                      n226 = property on="# to Average" class="DigNum (strict)"("Visible"=w407) -> ()  [unwired: 2 in, 2 out]
                      n227 = property on="Acquiring" class="DigNum (strict)"("Visible"=w407) -> ()  [unwired: 2 in, 2 out]
                      n228 = property on="Frame Mode" class="Ring (strict)"("Visible"=w408) -> ()  [unwired: 2 in, 2 out]
                      n229 = property on="Frames" class="DigNum (strict)"("Visible"=w408) -> ()  [unwired: 2 in, 2 out]
                    }
                  }
                  n230 = property on="Acq Mode" class="Enum (strict)"("Visible"=w391) -> ()  [unwired: 2 in, 2 out]
                  n231 = property on="Acq 1 Type" class="Ring (strict)"("Visible"=w391) -> ()  [unwired: 2 in, 2 out]
                }
              }
            }
            event "Perform Function": Value Change {
              n232 = event-data() -> ("NewVal"=w414:bool)  [unwired: 1 in, 3 out]
              n233 = case shown="True" w414 {
                tunnel: w415 -> [_ w418]
                frame False {
                }
                frame True {
                  n234 = while {
                    shift-left: 1 -> [w422]
                    shift-right: [w421] -> _
                    tunnel: "Function" -> [w419]
                    tunnel: w418 -> [w423]
                    stop <- w420 continue-if-true
                    n235 = case shown="2" w422 {
                      tunnel: w423 -> [_ w438 w469 _]
                      selector: w422 -> [_ w437 w468 w530]
                      tunnel: [0 w429 w467 w530] -> w421
                      tunnel: [FALSE TRUE TRUE w531] -> w420
                      tunnel: w419 -> [_ w428 w465 _]
                      frame 0, Default {
                        # "Error"
                        n236 = local write "Perform Function"(FALSE ("Retrieve Im 1")) -> ()
                      }
                      frame 1 {
                        n237 = case shown="\"Get Camera Status\", Default" w428 {
                          tunnel: [w444 w447 w451 w455] -> w440
                          frame "Get Camera Status", Default {
                            n238 = call "Create Command Packet 3.vi"("Camera ID (1)"=u8 1 ("Camera ID"), "Function #"=u16 1011) -> ("Cmd Packet"=w444:string)  [unwired: 9 in]
                          }
                          frame "Get SI Image Settings" {
                            n239 = call "Create Command Packet 3.vi"("Camera ID (1)"=u8 1 ("Camera ID"), "Function #"=u16 1041) -> ("Cmd Packet"=w447:string)  [unwired: 9 in]
                          }
                          frame "Get Image 1 Header" {
                            n240 = call "Create Command Packet 3.vi"("Camera ID (1)"=u8 1 ("Camera ID"), "Buffer/Avg #/Frames"=u16 1 ("Buffer #"), "Function #"=u16 1024) -> ("Cmd Packet"=w451:string)  [unwired: 8 in]
                          }
                          frame "Get Image 2 Header" {
                            n241 = call "Create Command Packet 3.vi"("Camera ID (1)"=u8 1 ("Camera ID"), "Buffer/Avg #/Frames"=u16 2 ("Buffer #"), "Function #"=u16 1024) -> ("Cmd Packet"=w455:string)  [unwired: 8 in]
                          }
                        }
                        n242 = call "Flush TCP-IP Input Buffer.vi"("TCP/IP ID"=w438) -> ("TCP/IP ID Out"=w439:refnum<k5>)  [unwired: 4 in]
                        n243 = Increment(x=w437) -> (x+1=w430:i32)
                        n244 = call "Send TCP-IP Cmd and Get Ackn 3.vi"("TCP/IP ID In"=w439, "Cmd Packet"=w440) -> ("Read String"=w441:string, "Accepted Flag"=w431:bool, "error out"=w427:errorcluster)  [unwired: 7 in, 4 out]
                        n245 = local write "Read String"(w441) -> ()
                        n246 = local write "Error out"(w427) -> ()
                        n247 = case shown="True" w431 {
                          frame False {
                            n248 = One Button Dialog(message="The Command sent was not accepted by the Camera Server.") -> ()  [unwired: 1 in, 1 out]
                          }
                          frame True {
                          }
                        }
                        n249 = Unbundle By Name(w427) -> ("status"=w432:bool)
                        n250 = Not(x=w431) -> (.not. x?=w435:bool)
                        n251 = Or(x=w435, y=w432) -> (x .or. y?=w434:bool)
                        n252 = Select(t=0, s=w434, f=w430) -> (s? t:f=w429:i32)
                      }
                      frame 2 {
                        # "Packet ID"
                        n253 = Increment(x=w468) -> (x+1=w467:i32)
                        n254 = call "Parse TCP-IP Response 4.vi"("TCP/IP ID"=w469) -> ("Header"=w460:string, "Packet ID"=w464:u8, "Command Done"=w463:cluster{"Function #":u16}, "Acq. Status"=w462:T5, "Image Packet"=w459:T6, "Status Array"=w458:sgl[], "SI Image Settings"=w457:T7, "error out"=w461:errorcluster)  [unwired: 4 in, 3 out]
                        n255 = case shown="No Error" w461 {
                          selector: w461 -> [_ w528]
                          tunnel: w464 -> [w477 _]
                          tunnel: w463 -> [w476 _]
                          tunnel: w462 -> [w475 _]
                          tunnel: w460 -> [w474 _]
                          tunnel: w459 -> [w473 _]
                          tunnel: w465 -> [w472 _]
                          tunnel: w458 -> [w471 _]
                          tunnel: w457 -> [w470 _]
                          frame No Error {
                            n256 = case shown="131" w477 {
                              tunnel: w476 -> [_ _]
                              tunnel: w475 -> [_ _]
                              tunnel: w474 -> [_ w479]
                              tunnel: w473 -> [_ _]
                              tunnel: w472 -> [_ w481]
                              tunnel: w471 -> [_ w480]
                              tunnel: w470 -> [_ w478]
                              frame 0, Default {
                              }
                              frame 131 {
                                # "Data Packet"
                                n257 = case shown="\"Get Camera Status\", Default" w481 {
                                tunnel: w480 -> [_ w525 _ _]
                                tunnel: w479 -> [_ _ w526 w527]
                                tunnel: w478 -> [w499 _ _ _]
                                frame "Get SI Image Settings" {
                                n258 = Unbundle By Name(w499) -> ("Exp. Time"=w491:u32, "# of Modes"=w487:u8, "Mode #"=w486:u8, "Avg N Images"=w484:u32, "Frames"=w483:u32, "Acq. Mode"=w482:u16, "Acq. Type"=w488:u16, "Serial Origin"=w498:i32, "Serial Length"=w497:i32, "Serial Binning"=w496:i32, "Parallel Origin"=w495:i32, "Parallel Length"=w494:i32, "Parallel Binning"=w493:i32)
                                n259 = case shown="0, Default" w482 {
                                frame 0, Default {
                                w500 = FALSE ("Visible")
                                n260 = Build Array("Acquire Image 1", "Stop Acquisition", "Acquire Image 1", "Stop Acquisition") -> (w501:string[])
                                n261 = property on="Acquire" class="Bool (strict)"("Strings [4]"=w501) -> ()  [unwired: 2 in, 2 out]
                                n262 = property on="# to Average" class="DigNum (strict)"("Visible"=w500) -> ()  [unwired: 2 in, 2 out]
                                n263 = property on="Acquiring" class="DigNum (strict)"("Visible"=w500) -> ()  [unwired: 2 in, 2 out]
                                n264 = property on="Frames" class="DigNum (strict)"("Visible"=w500) -> ()  [unwired: 2 in, 2 out]
                                n265 = property on="Frame Mode" class="Ring (strict)"("Visible"=w500) -> ()  [unwired: 2 in, 2 out]
                                }
                                frame 1 {
                                w506 = TRUE ("Visible")
                                w507 = FALSE ("Visible")
                                n266 = Build Array("Acquire Average", "Stop Acquisition", "Acquire Average", "Stop Acquisition") -> (w508:string[])
                                n267 = property on="Acquire" class="Bool (strict)"("Strings [4]"=w508) -> ()  [unwired: 2 in, 2 out]
                                n268 = property on="# to Average" class="DigNum (strict)"("Visible"=w506) -> ()  [unwired: 2 in, 2 out]
                                n269 = property on="Acquiring" class="DigNum (strict)"("Visible"=w506) -> ()  [unwired: 2 in, 2 out]
                                n270 = property on="Frames" class="DigNum (strict)"("Visible"=w507) -> ()  [unwired: 2 in, 2 out]
                                n271 = property on="Frame Mode" class="Ring (strict)"("Visible"=w507) -> ()  [unwired: 2 in, 2 out]
                                }
                                frame 2 {
                                w513 = FALSE ("Visible")
                                w514 = TRUE ("Visible")
                                n272 = Build Array("Acquire Frames", "Stop Acquisition", "Acquire Frames", "Stop Acquisition") -> (w515:string[])
                                n273 = property on="Acquire" class="Bool (strict)"("Strings [4]"=w515) -> ()  [unwired: 2 in, 2 out]
                                n274 = property on="# to Average" class="DigNum (strict)"("Visible"=w513) -> ()  [unwired: 2 in, 2 out]
                                n275 = property on="Acquiring" class="DigNum (strict)"("Visible"=w513) -> ()  [unwired: 2 in, 2 out]
                                n276 = property on="Frames" class="DigNum (strict)"("Visible"=w514) -> ()  [unwired: 2 in, 2 out]
                                n277 = property on="Frame Mode" class="Ring (strict)"("Visible"=w514) -> ()  [unwired: 2 in, 2 out]
                                }
                                }
                                n278 = for {
                                N: w487 -> [_]
                                tunnel: [w520] -> w485 mode=indexing
                                i -> [w523]
                                n279 = Format Into String(format string="%d", initial string="Mode ", w523) -> (resulting string=w520:string)  [unwired: 1 in, 1 out]
                                }
                                n280 = Bundle("Serial Origin"=w498, "Serial Length"=w497, "Serial Binning"=w496, "Parallel Origin"=w495, "Parallel Length"=w494, "Parallel Binning"=w493) -> (w492:T8)  [unwired: 1 in]
                                n281 = Divide(x=w491, y=1000.0 ("x/y")) -> (x/y=w489:dbl)
                                n282 = local write "Exposure Time"(w489) -> ()
                                n283 = local write "CCD Format Parameters"(w492) -> ()
                                n284 = local write "Acq Mode"(w482) -> ()
                                n285 = local write "Acq 1 Type"(w488) -> ()
                                n286 = local write "# to Average"(w484) -> ()
                                n287 = local write "Frames"(w483) -> ()
                                n288 = property on="Readout Mode" class="Ring (strict)"("Strings []"=w485, "Value"=w486) -> ()  [unwired: 2 in, 2 out]
                                }
                                frame "Get Camera Status", Default {
                                n289 = local read "index 1"() -> (w524:i32)
                                n290 = property on="index 1" class="DigNum (strict)"("Value (Signaling)"=w524) -> ()  [unwired: 2 in, 2 out]
                                "Camera Status [ ]" <- w525
                                }
                                frame "Get Image 1 Header" {
                                "Image Header" <- w526
                                }
                                frame "Get Image 2 Header" {
                                n291 = local write "Image Header"(w527) -> ()
                                }
                                }
                              }
                            }
                          }
                          frame Error {
                            n292 = local write "Error out"(w528) -> ()
                            n293 = call <vilib>:"Simple Error Handler.vi"("error source (\" \")"="There was an error in a TCP/IP read during an Image Acquisition.", "error in (no error)"=w528) -> ()  [unwired: 3 in, 5 out]
                          }
                        }
                      }
                      frame 3 {
                        w531 = FALSE ("Retrieve Im 1")
                        n294 = local write "Perform Function"(w531) -> ()
                      }
                    }
                  }
                }
              }
            }
            event "index 1", "index 2", "index 3": Value Change {
              # "Note that the indexes used below are not valid for all cameras.  Check the .cfg file for correct indexes."
              n295 = event-data() -> ()  [unwired: 1 in, 6 out]
              n296 = local read "Camera Status [ ]"() -> (w532:sgl[])
              n297 = Index Array(array=w532, index #1="index 1", index #2="index 2", index #3="index 3") -> (element #1=→"CCD Temp.":sgl, element #2=→"Backplate Temp.":sgl, element #3=→"Vacuum Pressure":sgl)
            }
            event "Display Style": Value Change {
              n298 = event-data() -> ("NewVal"=w539:i32)  [unwired: 1 in, 5 out]
              n299 = property on="Read String" class="Str"("Display Style"=w539) -> ()  [unwired: 2 in, 2 out]
            }
          }
        }
        "Error out" <- w13
        n300 = call "No EOC Error.vi"("error in"=w13) -> ("error out"=w15:errorcluster)  [unwired: 4 in]
        n301 = TCP Close Connection(connection ID=w14, error in (no error)=w15) -> ()  [unwired: 1 in, 2 out]
        n302 = call <vilib>:"General Error Handler.vi"("type of dialog (OK msg:1)"=w18, "error in (no error)"=w13) -> ()  [unwired: 9 in, 5 out]
        n303 = flat-sequence {
          frame #0 {
            n304 = local write "Function"(T4."Get SI Image Settings" ("Function")) -> ()
          }
          frame #1 {
            n305 = property on="Perform Function" class="Bool (strict)"("Value (Signaling)"=TRUE) -> ()  [unwired: 2 in, 2 out]
          }
        }
      }
      frame Error {
        # "There is no \"server\" sending. wait until TCP/IP Open error is = 0."
        n306 = event shown="[1] \"Stop\": Value Change" {
          selector: _ -> [_ _]
          dyn-events: _ -> [_ _]
          timeout: 50 -> [_ _]
          tunnel: [_ w542] -> w540
          event Timeout {
            n307 = event-data() -> ()  [unwired: 1 in, 2 out]
          }
          event "Stop": Value Change {
            n308 = event-data() -> ("NewVal"=w542:bool)  [unwired: 1 in, 2 out]
            n309 = local write "Stop"(FALSE ("Stop")) -> ()
          }
        }
      }
    }
  }
